vi "Initialize Robot.vi"(8 "error in":errorcluster, 10 "HOME?":bool, 11 "Gantry in":refnum<class "Gantry.lvclass">) -> (0 "error out":errorcluster, 3 "Gantry out":refnum<class "Gantry.lvclass">)   [LabVIEW 2026, in "Gantry.lvclass"]
uses:
  Gantry.lvclass
  <instrlib>/Aerotech Automation1/Private/Connect Controller_Simple.vi
  <instrlib>/Aerotech Automation1/Aerotech Automation1.lvlib
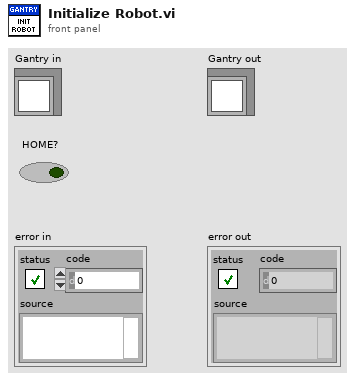
[diagram p1: front panel]
types:
  T1 = typedef "Virtual Modes.ctl" = enum16{"Nonvirtual", "Virtual"}
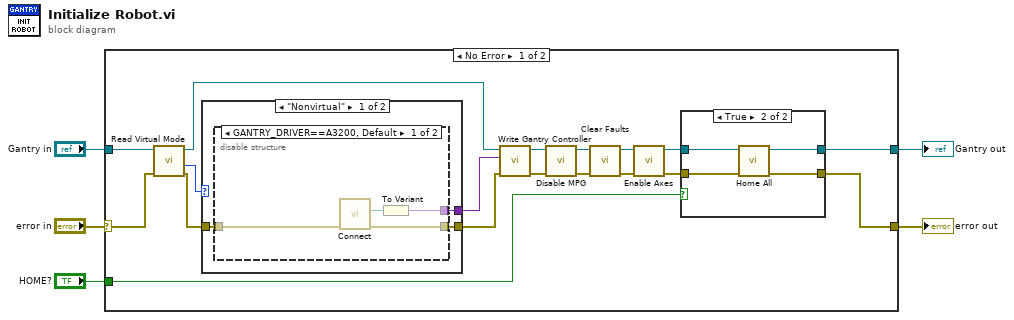
[diagram p0: block diagram]
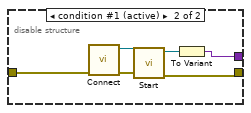
[diagram p2: hidden frame]
diagram:
  n1 = case shown="No Error" "error in" {
    selector: "error in" -> [w7 w45]
    tunnel: [w15 w45] -> w4
    tunnel: [w16 w44] -> w2
    tunnel: "Gantry in" -> [w8 w44]
    tunnel: "HOME?" -> [w19 _]
    frame No Error {
      n2 = call-dynamic "Read Virtual Mode.vi"("error in (no error)"=w7, "Gantry in"=w8) -> ("error out"=w9:errorcluster, "Virtual Mode"=w14:T1, "Gantry out"=w6:refnum<class "Gantry.lvclass">)  [unwired: 6 in, 1 out]
      n3 = case shown="\"Nonvirtual\"" w14 {
        tunnel: w9 -> [w26 w37]
        tunnel: [w25 w37] -> w12
        tunnel: [w24 _] -> w13
        frame "Nonvirtual" {
          n4 = disable-structure shown="GANTRY_DRIVER==A3200, Default" {
            disable-tunnel: w26 -> [w30 w32]
            disable-tunnel: [w29 w31] -> w25
            disable-tunnel: [w27 w33] -> w24
            frame condition #0 {
              n5 = call <instrlib>:"Connect.vi"("error in (no error)"=w30) -> ("error out"=w29:errorcluster, "controller"=w28:refnum<k24>)  [unwired: 9 in]
              n6 = To Variant(anything=w28) -> (Variant=w27:variant)
            }
            frame condition #1 (active) {
              n7 = call-poly <instrlib>:"Connect.vi"("error in (no error)"=w32) -> ("error out"=w35:errorcluster, "Controller Refnum out"=w36:refnum<k24>)  [unwired: 9 in]
              n8 = call <instrlib>:"Start.vi"("error in (no error)"=w35, "Controller Refnum in"=w36) -> ("error out"=w31:errorcluster, "Controller Refnum out"=w34:refnum<k24>)  [unwired: 8 in]
              n9 = To Variant(anything=w34) -> (Variant=w33:variant)
            }
          }
        }
        frame "Virtual" {
        }
      }
      n10 = call "Write Gantry Controller.vi"("error in (no error)"=w12, "Variant"=w13, "Gantry in"=w6) -> ("error out"=w11:errorcluster, "Gantry out"=w10:refnum<class "Gantry.lvclass">)  [unwired: 7 in]
      n11 = call-dynamic "Disable MPG.vi"("error in"=w11, "Gantry in"=w10) -> ("error out"=w20:errorcluster, "Gantry out"=w21:refnum<class "Gantry.lvclass">)  [unwired: 8 in]
      n12 = call-dynamic "Clear Faults.vi"("error in"=w20, "Gantry in"=w21) -> ("error out"=w23:errorcluster, "Gantry out"=w22:refnum<class "Gantry.lvclass">)  [unwired: 8 in]
      n13 = call-dynamic "Enable Axes.vi"("error in"=w23, "Gantry in"=w22) -> ("error out"=w18:errorcluster, "Gantry out"=w17:refnum<class "Gantry.lvclass">)  [unwired: 8 in]
      n14 = case shown="True" w19 {
        tunnel: w18 -> [w39 w42]
        tunnel: w17 -> [w38 w43]
        tunnel: [w38 w41] -> w16
        tunnel: [w39 w40] -> w15
        frame False {
        }
        frame True {
          n15 = call "Home All.vi"("error in (no error)"=w42, "Gantry in"=w43) -> ("error out"=w40:errorcluster, "Gantry out"=w41:refnum<class "Gantry.lvclass">)  [unwired: 8 in]
        }
      }
    }
    frame Error {
    }
  }
  "error out" <- w4
  "Gantry out" <- w2
